vi "OpenConnections.vi"(7 "process name":string, 8 "error in (no error)":errorcluster, 10 "Qbus":refnum<class "Qbus.lvclass">, 11 "config in":T1) -> (0 "error out":errorcluster, 3 "config out":T1)   [LabVIEW 2017, in "ModbusMaster.lvlib"]
uses:
  <vilib>/addons/InsightCM/Devices/Shared/Common/ModbusMaster/ModbusMaster.lvlib
  <vilib>/addons/InsightCM/Devices/Shared/Common/ModbusMaster/controls/config.ctl
  <vilib>/addons/InsightCM/Devices/Shared/Common/ModbusMaster/controls/ModbusDevice.ctl
  <vilib>/Modbus/master/Modbus Master.lvclass
  C:/Program Files (x86)/National Instruments/LabVIEW 2017/vi.lib/Modbus/subvis/Modbus API/Modbus API.lvclass
  <vilib>/addons/InsightCM/Devices/Shared/Common/ModbusMaster/controls/ModbusChannel.ctl
  <vilib>/addons/InsightCM/Devices/Shared/Common/ModbusMaster/controls/RegisterType.ctl
  <vilib>/addons/InsightCM/MessageBus/Base/controls/DataSource.ctl
  <vilib>/addons/InsightCM/MessageBus/Base/controls/KeyValuePair.ctl
  <vilib>/addons/Qbus/Qbus.lvclass
  <vilib>/Modbus/subvis/Modbus API/Modbus API.lvclass/Modbus API.ctl
  <vilib>/Modbus/subvis/Transmission Data Unit (ADU)/Transmission Data Unit/Transmission Data Unit.lvclass/Transmission Data Unit.ctl
  <vilib>/addons/TimerProcess/controls/taskType.ctl
  <vilib>/Modbus/master/Data Access/Read Timeout/Set Read Timeout.vi
  <vilib>/Modbus/subvis/Modbus API/Read Transmission Data Unit.vi
  <vilib>/Modbus/subvis/Modbus API/Write Transmission Data Unit.vi
  <vilib>/Modbus/subvis/Transmission Data Unit (ADU)/Transmission Data Unit/Data Access/timeouts/Write read operation timeout.vi
  <vilib>/addons/PointValueMap/subVIs/Point_Write_double.vi
  <vilib>/Modbus/subvis/Transmission Data Unit (ADU)/Transmission Data Unit/Transmission Data Unit.lvclass
  <vilib>/addons/InsightCM/Utilities/ChannelStatus/ChannelStatus.lvlib
  <vilib>/addons/TimerProcess/TimerProcess.lvlib
  <vilib>/addons/PointValueMap/PointValueMap.lvlib
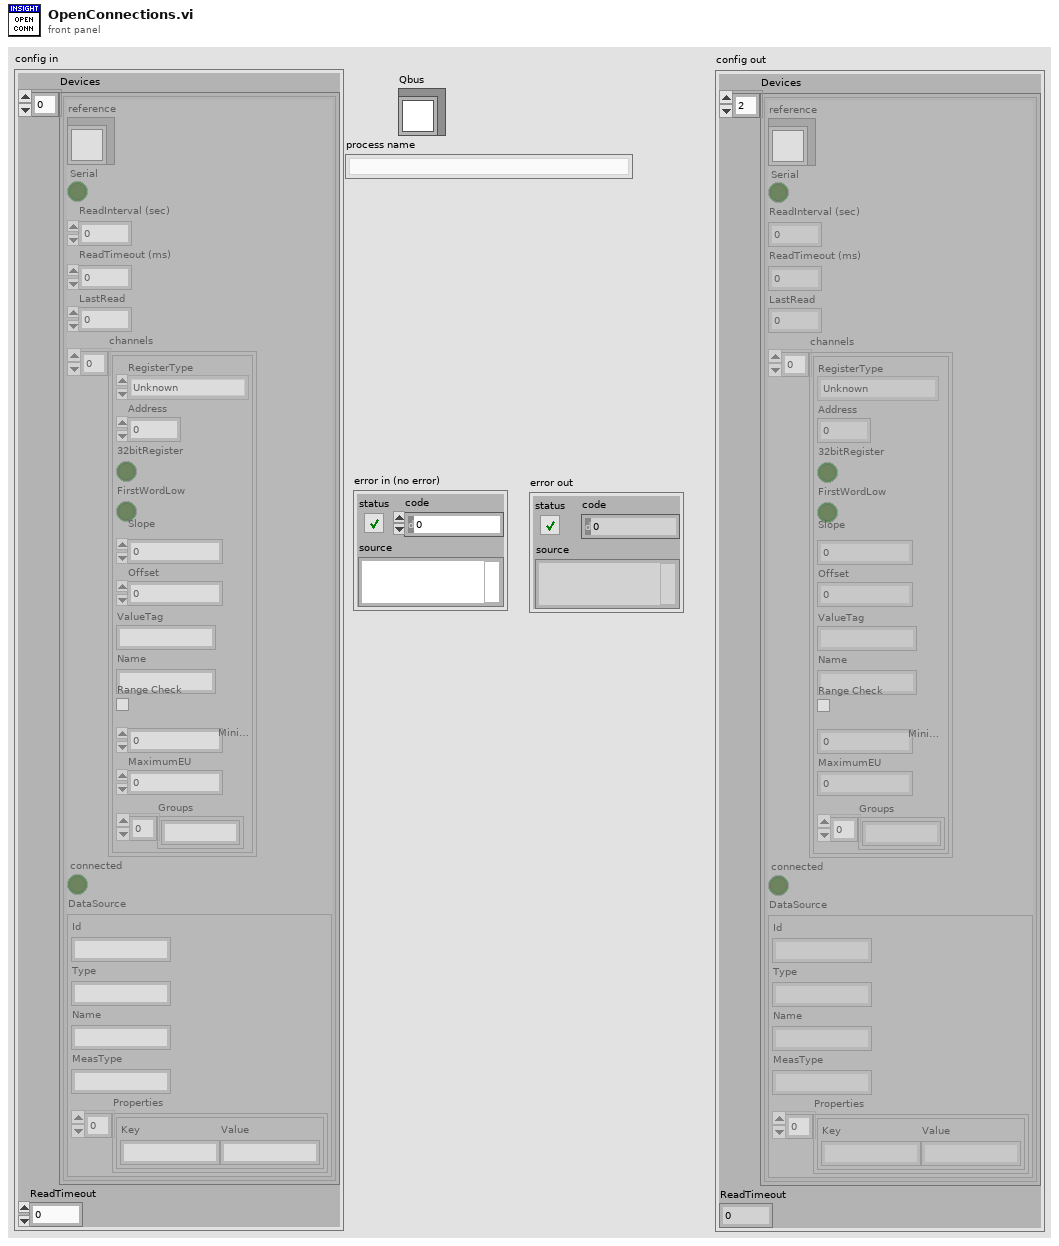
[diagram p1: front panel]
types:
  T1 = typedef "ModbusMaster.lvlib/config.ctl" = cluster{"Devices":T2[], "ReadTimeout":i32}
  T2 = typedef "ModbusMaster.lvlib/ModbusDevice.ctl" = cluster{"reference":refnum<class "Modbus Master.lvclass">, "Serial":bool, "ReadInterval (sec)":dbl, "ReadTimeout (ms)":i32, "LastRead":dbl, "channels":T3[], "connected":bool, "DataSource":T5}
  T3 = typedef "ModbusMaster.lvlib/ModbusChannel.ctl" = cluster{"RegisterType":T4, "Address":i32, "32bitRegister":bool, "FirstWordLow":bool, "Slope":dbl, "Offset":dbl, "ValueTag":string, "Name":string, "Range Check":bool, "MinimumEU":dbl, "MaximumEU":dbl, "Groups":string[]}
  T4 = typedef "ModbusMaster.lvlib/RegisterType.ctl" = enum16{"Unknown", "Coil", "Discrete Input", "Holding Register", "Input Register"}
  T5 = typedef "DataSource.ctl" = cluster{"Id":string, "Type":string, "Name":string, "MeasType":string, "Properties":T6[]}
  T6 = typedef "KeyValuePair.ctl" = cluster{"Key":string, "Value":string}
  T7 = typedef "TimerProcess.lvlib/taskType.ctl" = enum16{"single", "repeat"}
  T8 = typedef "PointValueMap.lvlib/PointMap.ctl" = refnum<data-value>
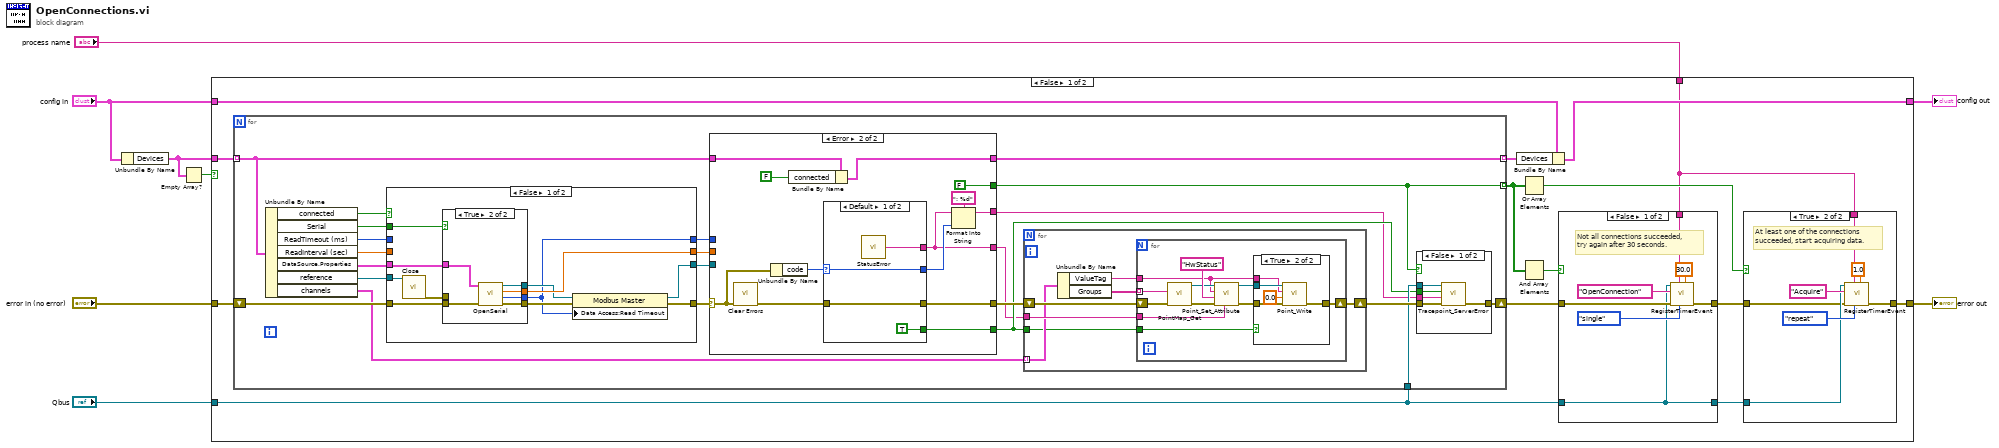
[diagram p0: block diagram]
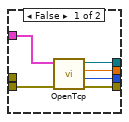
[diagram p5: hidden frame]
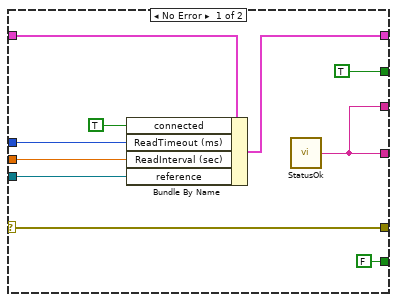
[diagram p7: hidden frame]
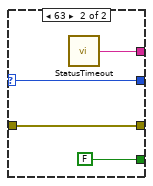
[diagram p8: hidden frame]
diagram:
  n1 = Unbundle By Name("config in") -> ("Devices"=w3:T2[])
  n2 = Empty Array?(array=w3) -> (empty?=w2:bool)
  n3 = case shown="False" w2 {
    tunnel: "config in" -> [w22 w150]
    tunnel: [w21 w150] -> w7
    tunnel: "error in (no error)" -> [w20 w151]
    tunnel: [w12 w151] -> w5
    tunnel: "Qbus" -> [w10 _]
    tunnel: w3 -> [w17 _]
    tunnel: "process name" -> [w9 _]
    frame False {
      n4 = for {
        tunnel: w17 -> [w39] mode=indexing
        shift-right: [w36] -> w19
        shift-left: w20 -> [w52]
        tunnel: [w44] -> w18 mode=indexing
        tunnel: [w31] -> w16 mode=indexing
        tunnel: w10 -> [w35]
        n5 = Unbundle By Name(w39) -> ("connected"=w41:bool, "Serial"=w40:bool, "ReadTimeout (ms)"=w42:i32, "ReadInterval (sec)"=w45:dbl, "DataSource.Properties"=w46:T6[], "reference"=w48:refnum<class "Modbus Master.lvclass">, "channels"=w38:T3[])
        n6 = case shown="False" w41 {
          tunnel: w46 -> [w93 _]
          tunnel: w52 -> [w92 w109]
          tunnel: [w91 w108] -> w51
          tunnel: [w90 w109] -> w50
          tunnel: [w88 w107] -> w49
          tunnel: w48 -> [w86 w107]
          tunnel: w45 -> [_ w108]
          tunnel: [w84 w106] -> w43
          tunnel: w42 -> [_ w106]
          tunnel: w40 -> [w83 _]
          frame False {
            n7 = call-dynamic "Close.vi"("Modbus master in"=w86) -> ("error out"=w85:errorcluster)  [unwired: 10 in]
            n8 = case shown="True" w83 {
              tunnel: w93 -> [w98 w105]
              tunnel: [w99 w104] -> w89
              tunnel: [w97 w103] -> w87
              tunnel: [w96 w102] -> w91
              tunnel: w92 -> [w95 w101]
              tunnel: w85 -> [_ _]
              tunnel: [w94 w100] -> w84
              frame False {
                n9 = call <vilib>:"OpenTcp.vi"("error in (no error)"=w95, "properties"=w98) -> ("error out"=w99:errorcluster, "read timeout (ms)"=w94:i32, "read interval (sec)"=w96:dbl, "serial master instance"=w97:refnum<class "Modbus Master.lvclass">)  [unwired: 6 in]
              }
              frame True {
                n10 = call <vilib>:"OpenSerial.vi"("error in (no error)"=w101, "properties"=w105) -> ("error out"=w104:errorcluster, "read timeout (ms)"=w100:i32, "read interval (sec)"=w102:dbl, "serial master instance"=w103:refnum<class "Modbus Master.lvclass">)  [unwired: 6 in]
              }
            }
            n11 = property class="Modbus Master"(reference=w87, error in=w89, "Data Access:Read Timeout"=w84) -> (reference out=w88:refnum<class "Modbus Master.lvclass">, error out=w90:errorcluster)
          }
          frame True {
          }
        }
        n12 = case shown="Error" w50 {
          selector: w50 -> [w117 w129]
          tunnel: [w110 w123] -> w33
          tunnel: w39 -> [w119 w131]
          tunnel: w51 -> [w118 _]
          tunnel: w49 -> [w115 _]
          tunnel: [w117 w125] -> w47
          tunnel: [w116 w128] -> w44
          tunnel: w43 -> [w114 _]
          tunnel: [TRUE ("connected") FALSE ("connected")] -> w31
          tunnel: [FALSE w126] -> w34
          tunnel: [w110 w120] -> w32
          frame No Error {
            n13 = Bundle By Name(cluster=w119, "connected"=TRUE, "ReadTimeout (ms)"=w114, "ReadInterval (sec)"=w118, "reference"=w115) -> (w116:T2)
            n14 = call <vilib>:"StatusOk.vi"() -> ("status"=w110:string)  [unwired: 5 in]
          }
          frame Error {
            n15 = call <vilib>:"Clear Errors.vi"("error in (no error)"=w129) -> ("error out"=w124:errorcluster)  [unwired: 5 in, 1 out]
            n16 = Unbundle By Name(w129) -> ("code"=w122:i32)
            n17 = Bundle By Name(cluster=w131, "connected"=FALSE) -> (w128:T2)
            n18 = case shown="Default" w122 {
              selector: w122 -> [w133 w138]
              tunnel: [TRUE FALSE] -> w126
              tunnel: [w135 w139] -> w125
              tunnel: w124 -> [w135 w139]
              tunnel: [w133 w138] -> w121
              tunnel: [w134 w137] -> w120
              frame Default {
                n19 = call <vilib>:"StatusError.vi"() -> ("status"=w134:string)  [unwired: 5 in]
              }
              frame 63 {
                n20 = call <vilib>:"StatusTimeout.vi"() -> ("status"=w137:string)  [unwired: 5 in]
              }
            }
            n21 = Format Into String(format string=": %d", initial string=w120, w121) -> (resulting string=w123:string)  [unwired: 1 in, 1 out]
          }
        }
        n22 = for {
          tunnel: w32 -> [w63]
          shift-right: [w61] -> w37
          shift-left: w47 -> [w64]
          tunnel: w38 -> [w62] mode=indexing
          tunnel: w34 -> [w59]
          n23 = Unbundle By Name(w62) -> ("ValueTag"=w60:string, "Groups"=w65:string[])
          n24 = for {
            tunnel: w65 -> [w76] mode=indexing
            tunnel: w63 -> [w73]
            tunnel: w60 -> [w67]
            tunnel: w59 -> [w66]
            shift-right: [w68] -> w61
            shift-left: w64 -> [w75]
            n25 = call <vilib>:"PointMap_Get.vi"("error in (no error)"=w75, "Name"=w76) -> ("error out"=w71:errorcluster, "Map Out"=w72:T8)  [unwired: 7 in, 1 out]
            n26 = call <vilib>:"Point_Set_Attribute.vi"("Value"=w73, "Error In"=w71, "Attribute"="HwStatus", "Tag"=w67, "Map"=w72) -> ("Error Out"=w69:errorcluster, "Map Out"=w70:T8)  [unwired: 5 in]
            n27 = case shown="True" w66 {
              tunnel: w70 -> [_ w82]
              tunnel: w69 -> [w77 w81]
              tunnel: [w77 w80] -> w68
              tunnel: w67 -> [_ w79]
              frame False {
              }
              frame True {
                n28 = call-poly <vilib>:"Point_Write.vi"("Error In"=w81, "Value"=0.0, "Tag"=w79, "Map"=w82) -> ("Error Out"=w80:errorcluster)  [unwired: 6 in, 1 out]
              }
            }
          }
        }
        n29 = case shown="False" w31 {
          tunnel: w37 -> [w57 w58]
          tunnel: [w56 w58] -> w36
          tunnel: w35 -> [w55 _]
          tunnel: w34 -> [w54 _]
          tunnel: w33 -> [w53 _]
          frame False {
            n30 = call <vilib>:"Tracepoint_ServerError.vi"("error in (no error)"=w57, "String"=w53, "Error"=w54, "Qbus"=w55) -> ("error out"=w56:errorcluster)  [unwired: 7 in]
          }
          frame True {
          }
        }
      }
      n31 = Bundle By Name(cluster=w22, "Devices"=w18) -> (w21:T1)
      n32 = Or Array Elements(Boolean array=w16) -> (logical OR=w11:bool)
      n33 = And Array Elements(Boolean array=w16) -> (logical AND=w15:bool)
      n34 = case shown="False" w15 {
        tunnel: w19 -> [w144 w149]
        tunnel: [w143 w149] -> w13
        tunnel: w10 -> [w142 w148]
        tunnel: [w142 w148] -> w14
        tunnel: w9 -> [w141 _]
        frame False {
          # "Not all connections succeeded,\ntry again after 30 seconds."
          n35 = call <vilib>:"RegisterTimerEvent.vi"("interval (sec)"=30.0, "type"=taskType."single", "process name"=w141, "error in (no error)"=w144, "callback action"="OpenConnection", "qbus in"=w142) -> ("error out"=w143:errorcluster)  [unwired: 4 in, 1 out]
        }
        frame True {
        }
      }
      n36 = case shown="True" w11 {
        tunnel: w13 -> [w23 w25]
        tunnel: [w23 w27] -> w12
        tunnel: w14 -> [_ w26]
        tunnel: w9 -> [_ w24]
        frame False {
        }
        frame True {
          # "At least one of the connections\nsucceeded, start acquiring data."
          n37 = call <vilib>:"RegisterTimerEvent.vi"("interval (sec)"=1.0, "type"=taskType."repeat", "process name"=w24, "error in (no error)"=w25, "callback action"="Acquire", "qbus in"=w26) -> ("error out"=w27:errorcluster)  [unwired: 4 in, 1 out]
        }
      }
    }
    frame True {
    }
  }
  "config out" <- w7
  "error out" <- w5
